vi "Obtain Semaphore.vi"(8 "error in":errorcluster, 11 "Serial IO in":refnum<class "Serial IO.lvclass">) -> (0 "error out":errorcluster, 3 "Serial IO out":refnum<class "Serial IO.lvclass">)   [LabVIEW 2015, in "Serial IO.lvclass"]
doc: "Obtain a reference to a semaphore for preventing communication clashes when classes are accessed in different loops. The reference will be unique to the instance of the SerialIO object."
uses:
  Serial IO.lvclass
  Serial IO.lvclass/Serial IO.ctl
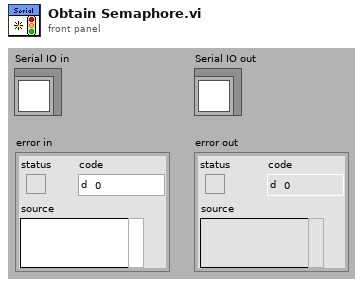
[diagram p1: front panel]
types:
  T1 = typedef "Semaphore RefNum" = refnum<k1>
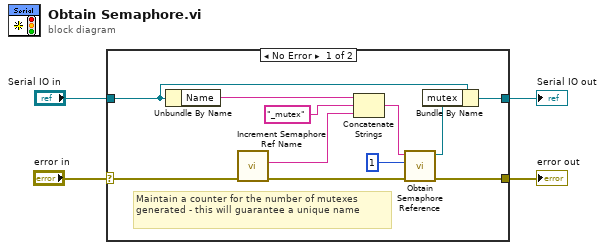
[diagram p0: block diagram]
diagram:
  n1 = case shown="No Error" "error in" {
    selector: "error in" -> [w6 w17]
    tunnel: [w14 w17] -> w3
    tunnel: [w13 w16] -> w1
    tunnel: "Serial IO in" -> [w8 w16]
    frame No Error {
      # "Maintain a counter for the number of mutexes generated - this will guarantee a unique name"
      n2 = Unbundle By Name(w8) -> ("Name"=w11:string)
      n3 = call "Increment Semaphore Ref Name.vi"("error in"=w6) -> ("error out"=w5:errorcluster, "appendStr"=w7:string)  [unwired: 9 in]
      n4 = Concatenate Strings(w11, "_mutex", w7) -> (w12:string)
      n5 = call <vilib>:"Obtain Semaphore Reference.vi"("error in (no error)"=w5, "size (1)"=1, "name (unnamed)"=w12) -> ("error out"=w14:errorcluster, "semaphore"=w15:T1)  [unwired: 2 in, 1 out]
      n6 = Bundle By Name(cluster=w8, "mutex"=w15) -> (w13:refnum<class "Serial IO.lvclass">)
    }
    frame Error {
    }
  }
  "error out" <- w3
  "Serial IO out" <- w1
